vi "stage_dither.vi"(8 "error in (no error)":errorcluster, 9 "Data":variant, 10 "Stage Name":string, 11 "newport_xps in":refnum<class "newport_xps.lvclass">) -> (0 "error out":errorcluster, 3 "newport_xps out":refnum<class "newport_xps.lvclass">)   [LabVIEW 2015, in "newport_xps.lvclass"]
uses:
  newport_xps.lvclass
  newport_xps.lvclass/newport_xps.ctl
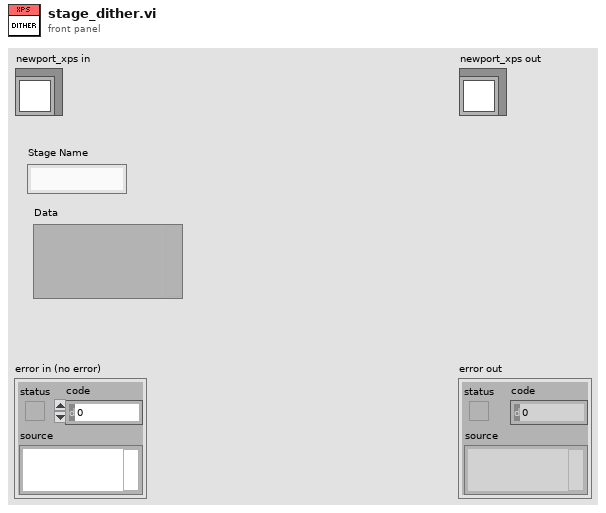
[diagram p1: front panel]
types:
  T1 = cluster{"connection TCP":refnum<k5>, "LogTo File":bool, "Log File refnum":refnum<file>, "no error if error log":bool}
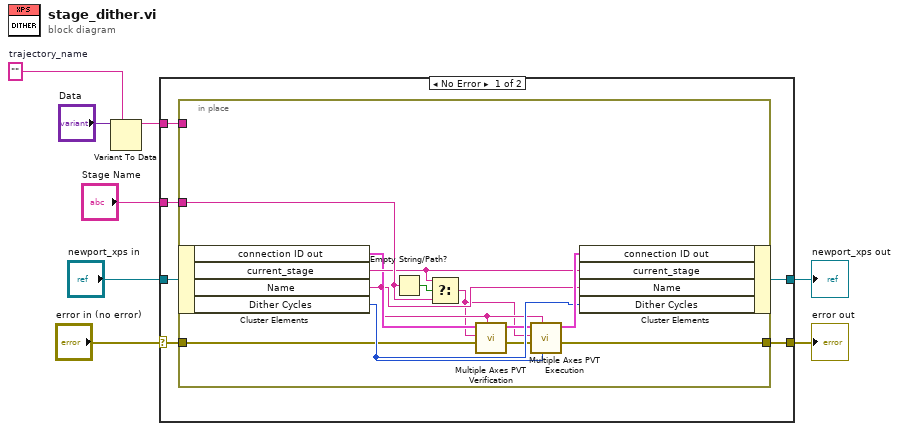
[diagram p0: block diagram]
diagram:
  w5 = ""  # trajectory_name
  n1 = Variant To Data(type=w5, Variant="Data") -> (data=w3:string)  [unwired: 1 in, 1 out]
  n2 = case shown="No Error" "error in (no error)" {
    selector: "error in (no error)" -> [w11 w28]
    tunnel: "newport_xps in" -> [w14 w27]
    tunnel: "Stage Name" -> [w13 _]
    tunnel: w3 -> [w12 _]
    tunnel: [w10 w28] -> w2
    tunnel: [w9 w27] -> w1
    frame No Error {
      n3 = in-place {
        in-place-border: w13 -> [w25]
        in-place-border: w12 -> [_]
        in-place-border: w11 -> [w20]
        in-place-border: [w23] -> w10
        n4 = in-place-cluster #1(w14) -> ("connection ID out"=w18:T1, "current_stage"=w21:string, "Name"=w16:string, "Dither Cycles"=w22:u32)
        n5 = Empty String/Path?(string/path=w25) -> (empty?=w26:bool)
        n6 = Select(t=w21, s=w26, f=w25) -> (s? t:f=w15:string)
        n7 = call "Multiple Axes PVT Verification.vi"("Trajectory File Name"=w16, "XPS error in (no error)"=w20, "MultipleAxes Group Name (250 c max)"=w15, "connection ID in"=w18) -> ("XPS error out"=w19:errorcluster, "connection ID out"=w17:T1)  [unwired: 5 in, 1 out]
        n8 = call "Multiple Axes PVT Execution.vi"("Execution Number"=w22, "Trajectory File Name"=w16, "XPS error in (no error)"=w19, "MultipleAxes Group Name (250 c max)"=w15, "connection ID in"=w17) -> ("XPS error out"=w23:errorcluster, "connection ID out"=w24:T1)  [unwired: 4 in, 1 out]
        n9 = in-place-cluster #1("connection ID out"=w24, "current_stage"=w21, "Name"=w16, "Dither Cycles"=w22) -> (w9:refnum<class "newport_xps.lvclass">)
      }
    }
    frame Error {
    }
  }
  "error out" <- w2
  "newport_xps out" <- w1
